vi "Control_iPS.vi"() -> ()   [LabVIEW 2015]
panel:
  out "Rate (T/min)":dbl
  out "Communication 3":string="\n"
  out "Communication 2":string="\n"
  out "Communication":string="\n"
  out "Switch Heater Status":string
  out "Switch Heater":bool
  out "Status Buttons":enum32{"HOLD", "To Set", "To Zero"}(radio)
  out "STATUS":string
  in  "Record new values":bool
  out "Field from current in leads (T)":dbl
  out "Real Field (T)":dbl
  out "Set Field (T)":dbl
  out "Helium Level (%)":dbl
  in  "error in (no error)":errorcluster
  out "error out":errorcluster
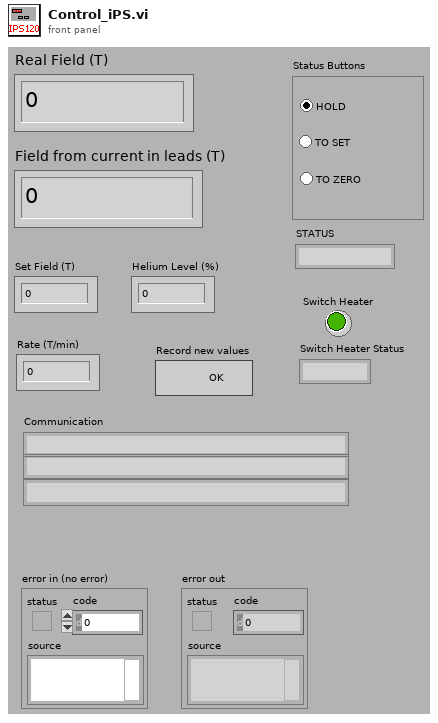
[diagram p1: front panel]
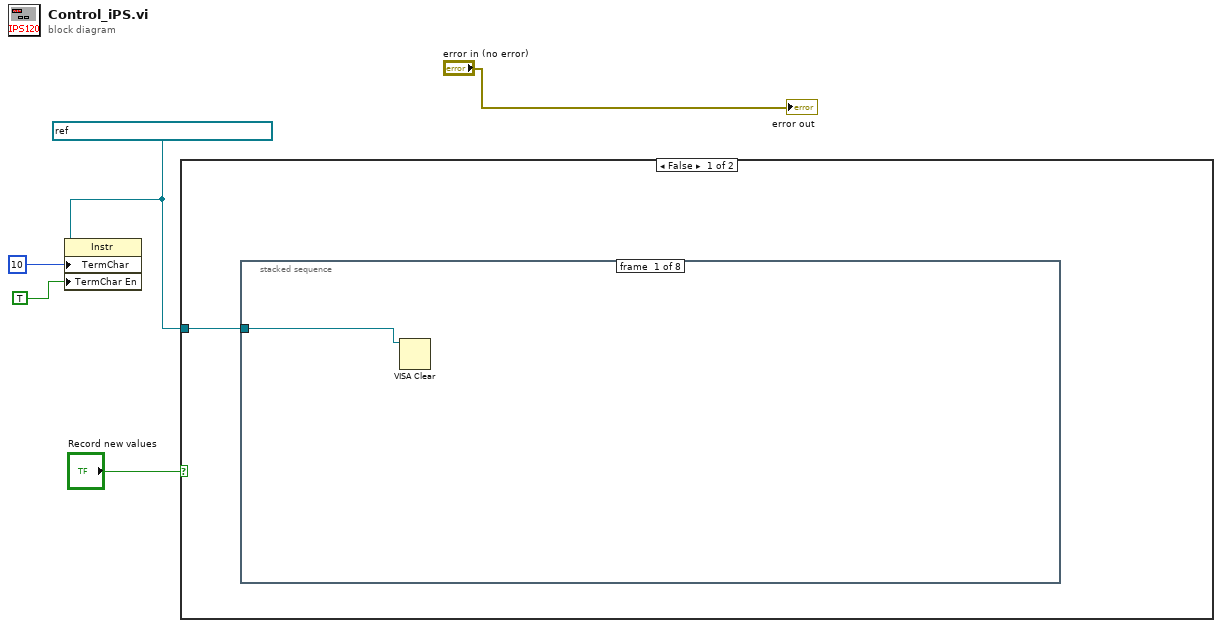
[diagram p0: block diagram]
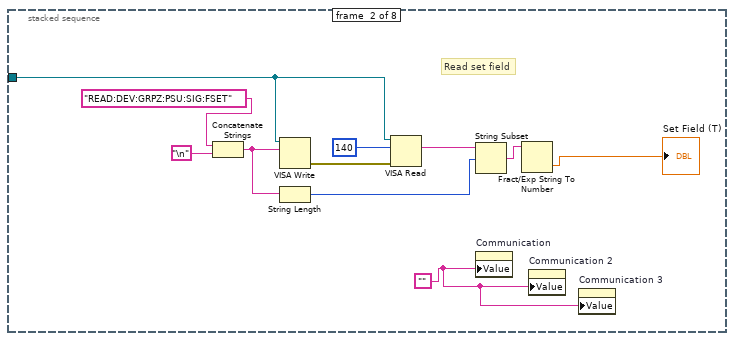
[diagram p2: hidden frame]
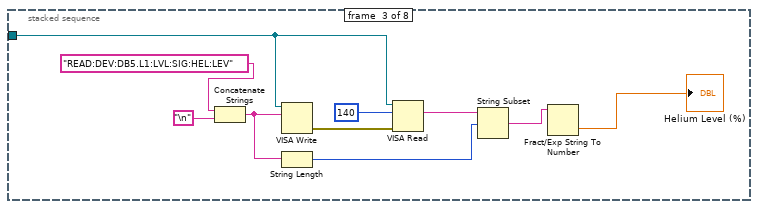
[diagram p3: hidden frame]
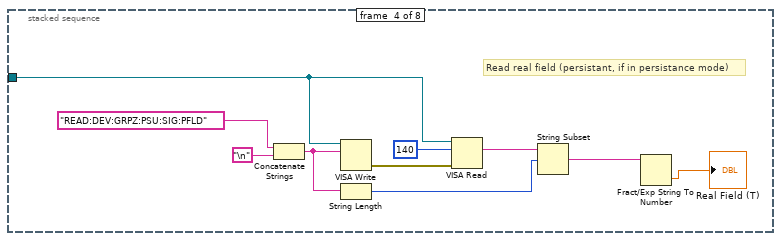
[diagram p4: hidden frame]
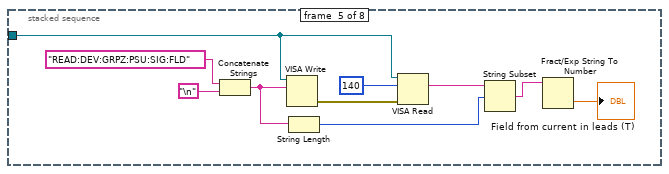
[diagram p5: hidden frame]
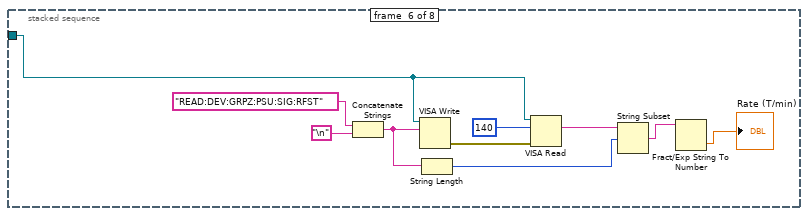
[diagram p6: hidden frame]
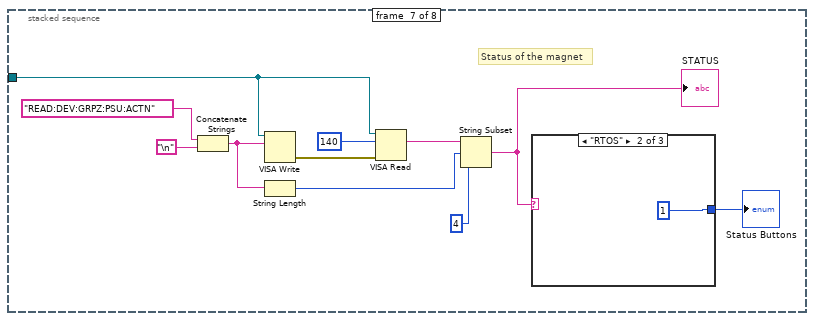
[diagram p7: hidden frame]
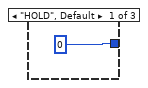
[diagram p8: hidden frame]
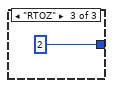
[diagram p9: hidden frame]
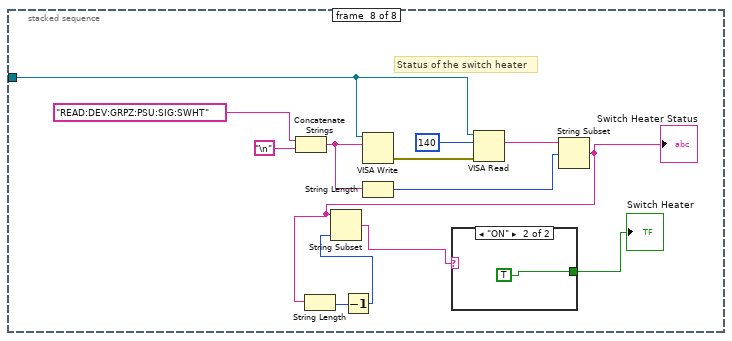
[diagram p10: hidden frame]
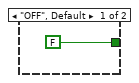
[diagram p11: hidden frame]
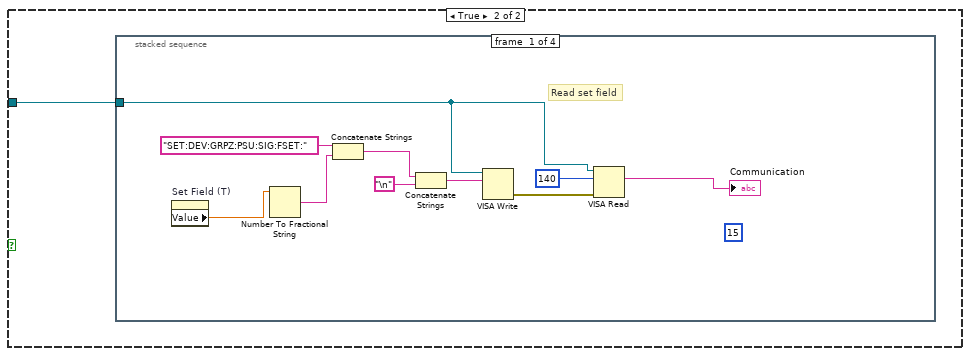
[diagram p12: hidden frame]
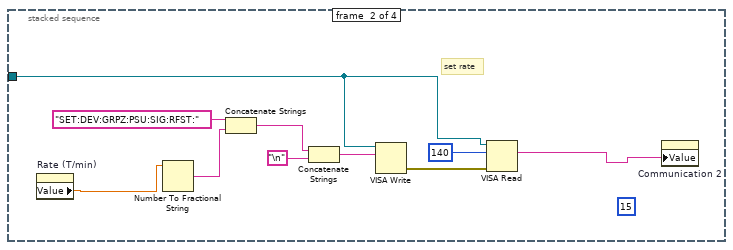
[diagram p13: hidden frame]
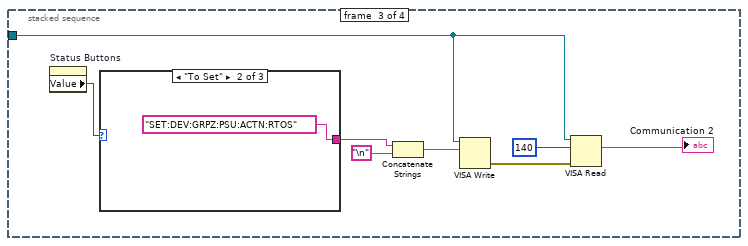
[diagram p14: hidden frame]
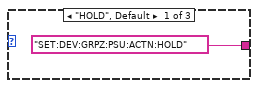
[diagram p15: hidden frame]
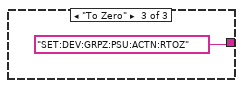
[diagram p16: hidden frame]
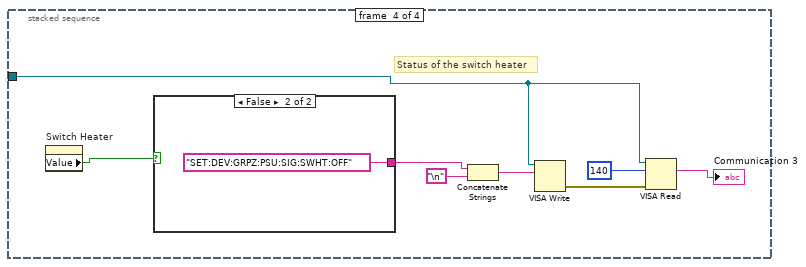
[diagram p17: hidden frame]
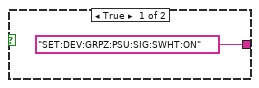
[diagram p18: hidden frame]
diagram:
  w2 = refnum<visa-resource-name> "TCPIP0::192.168.128.3::7020::SOCKET" ("VISA resource name")
  n1 = property class="Instr"(reference=w2, "TermChar"=10, "TermChar En"=TRUE) -> ()  [unwired: 1 in, 2 out]
  n2 = case shown="False" "Record new values" {
    tunnel: w2 -> [w6 w88]
    frame False {
      n3 = stacked-sequence {
        tunnel: w6 -> [w7 w9 w19 w29 w39 w50 w60 w77]
        frame #0 {
          n4 = VISA Clear(VISA resource name=w7) -> ()  [unwired: 1 in, 2 out]
        }
        frame #1 {
          w8 = ""
          # "Read set field"
          n5 = Concatenate Strings("READ:DEV:GRPZ:PSU:SIG:FSET" ("string"), "\n") -> (w11:string)
          n6 = VISA Write(VISA resource name=w9, write buffer=w11) -> (error out=w17:errorcluster)  [unwired: 1 in, 2 out]
          n7 = String Length(string=w11) -> (length=w12:i32)
          n8 = VISA Read(VISA resource name=w9, byte count=140, error in (no error)=w17) -> (read buffer=w13:string)  [unwired: 3 out]
          n9 = String Subset(string=w13, offset (0)=w12) -> (substring=w10:string)  [unwired: 1 in]
          n10 = property on="Communication" class="Str"("Value"=w8) -> ()  [unwired: 2 in, 2 out]
          n11 = Fract/Exp String To Number(string=w10) -> (number=→"Set Field (T)":dbl)  [unwired: 3 in, 1 out]
          n12 = property on="Communication 2" class="Str"("Value"=w8) -> ()  [unwired: 2 in, 2 out]
          n13 = property on="Communication 3" class="Str"("Value"=w8) -> ()  [unwired: 2 in, 2 out]
        }
        frame #2 {
          n14 = Concatenate Strings("READ:DEV:DB5.L1:LVL:SIG:HEL:LEV" ("string"), "\n") -> (w22:string)
          n15 = VISA Write(VISA resource name=w19, write buffer=w22) -> (error out=w28:errorcluster)  [unwired: 1 in, 2 out]
          n16 = String Length(string=w22) -> (length=w23:i32)
          n17 = VISA Read(VISA resource name=w19, byte count=140, error in (no error)=w28) -> (read buffer=w24:string)  [unwired: 3 out]
          n18 = String Subset(string=w24, offset (0)=w23) -> (substring=w21:string)  [unwired: 1 in]
          n19 = Fract/Exp String To Number(string=w21) -> (number=→"Helium Level (%)":dbl)  [unwired: 3 in, 1 out]
        }
        frame #3 {
          # "Read real field (persistant, if in persistance mode)"
          n20 = Concatenate Strings("READ:DEV:GRPZ:PSU:SIG:PFLD" ("string"), "\n") -> (w31:string)
          n21 = VISA Write(VISA resource name=w29, write buffer=w31) -> (error out=w37:errorcluster)  [unwired: 1 in, 2 out]
          n22 = String Length(string=w31) -> (length=w32:i32)
          n23 = VISA Read(VISA resource name=w29, byte count=140, error in (no error)=w37) -> (read buffer=w33:string)  [unwired: 3 out]
          n24 = String Subset(string=w33, offset (0)=w32) -> (substring=w30:string)  [unwired: 1 in]
          n25 = Fract/Exp String To Number(string=w30) -> (number=→"Real Field (T)":dbl)  [unwired: 3 in, 1 out]
        }
        frame #4 {
          n26 = Concatenate Strings("READ:DEV:GRPZ:PSU:SIG:FLD" ("string"), "\n") -> (w43:string)
          n27 = VISA Write(VISA resource name=w39, write buffer=w43) -> (error out=w47:errorcluster)  [unwired: 1 in, 2 out]
          n28 = String Length(string=w43) -> (length=w41:i32)
          n29 = VISA Read(VISA resource name=w39, byte count=140, error in (no error)=w47) -> (read buffer=w42:string)  [unwired: 3 out]
          n30 = String Subset(string=w42, offset (0)=w41) -> (substring=w40:string)  [unwired: 1 in]
          n31 = Fract/Exp String To Number(string=w40) -> (number=→"Field from current in leads (T)":dbl)  [unwired: 3 in, 1 out]
        }
        frame #5 {
          n32 = Concatenate Strings("READ:DEV:GRPZ:PSU:SIG:RFST" ("string"), "\n") -> (w54:string)
          n33 = VISA Write(VISA resource name=w50, write buffer=w54) -> (error out=w58:errorcluster)  [unwired: 1 in, 2 out]
          n34 = String Length(string=w54) -> (length=w52:i32)
          n35 = VISA Read(VISA resource name=w50, byte count=140, error in (no error)=w58) -> (read buffer=w53:string)  [unwired: 3 out]
          n36 = String Subset(string=w53, offset (0)=w52) -> (substring=w51:string)  [unwired: 1 in]
          n37 = Fract/Exp String To Number(string=w51) -> (number=→"Rate (T/min)":dbl)  [unwired: 3 in, 1 out]
        }
        frame #6 {
          # "Status of the magnet"
          n38 = Concatenate Strings("READ:DEV:GRPZ:PSU:ACTN" ("string"), "\n") -> (w63:string)
          n39 = VISA Write(VISA resource name=w60, write buffer=w63) -> (error out=w69:errorcluster)  [unwired: 1 in, 2 out]
          n40 = String Length(string=w63) -> (length=w64:i32)
          n41 = VISA Read(VISA resource name=w60, byte count=140, error in (no error)=w69) -> (read buffer=w65:string)  [unwired: 3 out]
          n42 = String Subset(string=w65, offset (0)=w64, length (rest)=4) -> (substring=w62:string)
          "STATUS" <- w62
          n43 = case shown="\"RTOS\"" w62 {
            tunnel: [0 1 2] -> w61
            frame "HOLD", Default {
            }
            frame "RTOS" {
            }
            frame "RTOZ" {
            }
          }
          "Status Buttons" <- w61
        }
        frame #7 {
          # "Status of the switch heater"
          n44 = Concatenate Strings("READ:DEV:GRPZ:PSU:SIG:SWHT" ("string"), "\n") -> (w79:string)
          n45 = VISA Write(VISA resource name=w77, write buffer=w79) -> (error out=w85:errorcluster)  [unwired: 1 in, 2 out]
          n46 = String Length(string=w79) -> (length=w80:i32)
          n47 = VISA Read(VISA resource name=w77, byte count=140, error in (no error)=w85) -> (read buffer=w81:string)  [unwired: 3 out]
          n48 = String Subset(string=w81, offset (0)=w80) -> (substring=w73:string)  [unwired: 1 in]
          "Switch Heater Status" <- w73
          n49 = String Length(string=w73) -> (length=w76:i32)
          n50 = Decrement(x=w76) -> (x-1=w75:i32)
          n51 = String Subset(string=w73, length (rest)=w75) -> (substring=w74:string)  [unwired: 1 in]
          n52 = case shown="\"ON\"" w74 {
            tunnel: [FALSE TRUE] -> w78
            frame "OFF", Default {
            }
            frame "ON" {
            }
          }
          "Switch Heater" <- w78
        }
      }
    }
    frame True {
      n53 = stacked-sequence {
        tunnel: w88 -> [w90 w101 w110 w121]
        frame #0 {
          (unwired) 15
          # "Read set field"
          n54 = property on="Set Field (T)" class="DigNum (strict)"() -> ("Value"=w91:dbl)  [unwired: 2 in, 2 out]
          n55 = Number To Fractional String(number=w91) -> (F-format string=w97:string)  [unwired: 3 in]
          n56 = Concatenate Strings("SET:DEV:GRPZ:PSU:SIG:FSET:" ("string"), w97) -> (w92:string)
          n57 = Concatenate Strings(w92, "\n") -> (w93:string)
          n58 = VISA Write(VISA resource name=w90, write buffer=w93) -> (error out=w96:errorcluster)  [unwired: 1 in, 2 out]
          n59 = VISA Read(VISA resource name=w90, byte count=140, error in (no error)=w96) -> (read buffer=→"Communication":string)  [unwired: 3 out]
        }
        frame #1 {
          (unwired) 15
          # "set rate"
          n60 = property on="Rate (T/min)" class="DigNum (strict)"() -> ("Value"=w100:dbl)  [unwired: 2 in, 2 out]
          n61 = Number To Fractional String(number=w100) -> (F-format string=w107:string)  [unwired: 3 in]
          n62 = Concatenate Strings("SET:DEV:GRPZ:PSU:SIG:RFST:" ("string"), w107) -> (w102:string)
          n63 = Concatenate Strings(w102, "\n") -> (w103:string)
          n64 = VISA Write(VISA resource name=w101, write buffer=w103) -> (error out=w106:errorcluster)  [unwired: 1 in, 2 out]
          n65 = VISA Read(VISA resource name=w101, byte count=140, error in (no error)=w106) -> (read buffer=w99:string)  [unwired: 3 out]
          n66 = property on="Communication 2" class="Str"("Value"=w99) -> ()  [unwired: 2 in, 2 out]
        }
        frame #2 {
          n67 = property on="Status Buttons" class="RadioBtnsControl (strict)"() -> ("Value"=w111:enum32{"HOLD", "To Set", "To Zero"})  [unwired: 2 in, 2 out]
          n68 = case shown="\"To Set\"" w111 {
            tunnel: ["SET:DEV:GRPZ:PSU:ACTN:HOLD" ("string") "SET:DEV:GRPZ:PSU:ACTN:RTOS" ("string") "SET:DEV:GRPZ:PSU:ACTN:RTOZ" ("string")] -> w112
            frame "HOLD", Default {
            }
            frame "To Set" {
            }
            frame "To Zero" {
            }
          }
          n69 = Concatenate Strings(w112, "\n") -> (w113:string)
          n70 = VISA Write(VISA resource name=w110, write buffer=w113) -> (error out=w116:errorcluster)  [unwired: 1 in, 2 out]
          n71 = VISA Read(VISA resource name=w110, byte count=140, error in (no error)=w116) -> (read buffer=→"Communication 2":string)  [unwired: 3 out]
        }
        frame #3 {
          # "Status of the switch heater"
          n72 = property on="Switch Heater" class="Bool (strict)"() -> ("Value"=w122:bool)  [unwired: 2 in, 2 out]
          n73 = case shown="False" w122 {
            tunnel: ["SET:DEV:GRPZ:PSU:SIG:SWHT:ON" ("string") "SET:DEV:GRPZ:PSU:SIG:SWHT:OFF" ("string")] -> w123
            frame True {
            }
            frame False {
            }
          }
          n74 = Concatenate Strings(w123, "\n") -> (w124:string)
          n75 = VISA Write(VISA resource name=w121, write buffer=w124) -> (error out=w127:errorcluster)  [unwired: 1 in, 2 out]
          n76 = VISA Read(VISA resource name=w121, byte count=140, error in (no error)=w127) -> (read buffer=→"Communication 3":string)  [unwired: 3 out]
        }
      }
    }
  }
  "error out" <- "error in (no error)"
